vi "18_TimeTaggerNetwork_server.vi"(8 "error in (no error)":errorcluster) -> (0 "error out":errorcluster)   [LabVIEW 2014]
uses:
  SwabianInstruments.TimeTagger
panel:
  out "log messages":string
  out "test signal":bool[](array[boolean])
  out "Counter measurement":i32[][](graph)
  in  "stop":bool
  # "Run the program to set up a server on default port 41101.\n\nThis VI will switch on and off the internal test-signal on channels 1-4\nin a cyclic pattern. \n\nYou can use the VI 18_TimeTaggerNetwork_client.vi to connect to this\nserver and to repeat the measurement on the client side."
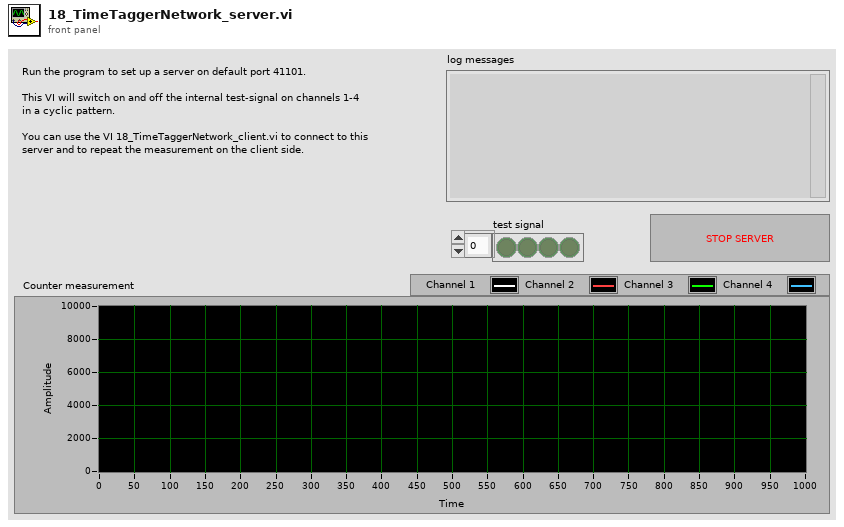
[diagram p1: front panel]
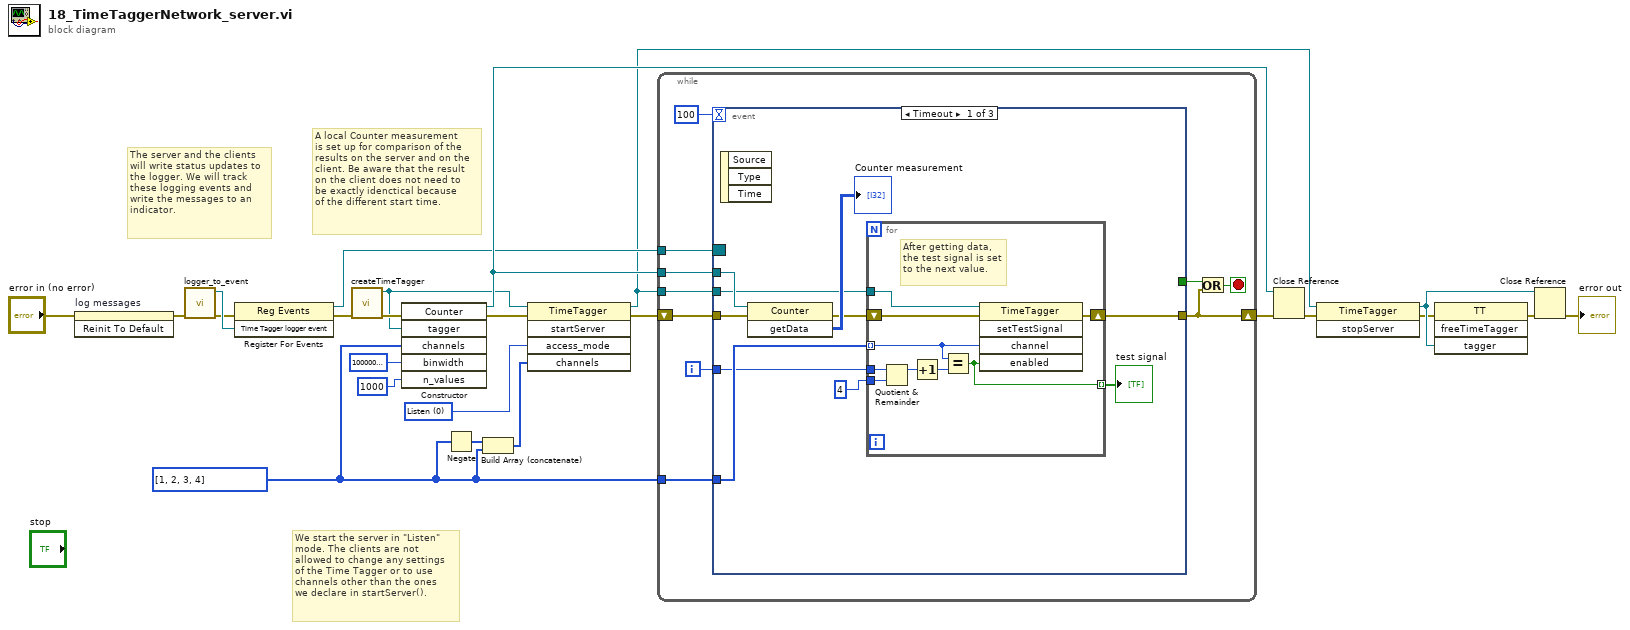
[diagram p0: block diagram]
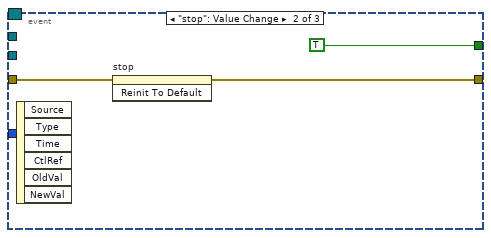
[diagram p2: hidden frame]
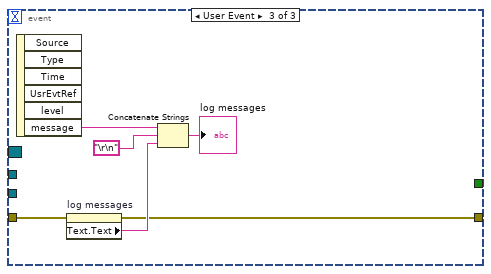
[diagram p3: hidden frame]
diagram:
  w14 = 0 items=["Listen", "Synchronous", "Control", "SynchronousControl"] ("access")
  w2 = i32[] [1, 2, 3, 4] ("channel")
  # "A local Counter measurement\nis set up for comparison of the\nresults on the server and on the\nclient. Be aware that the result\non the client does not need to\nbe exactly idenctical because\nof the different start time."
  # "The server and the clients\nwill write status updates to\nthe logger. We will track\nthese logging events and\nwrite the messages to an\nindicator."
  # "We start the server in \"Listen\"\nmode. The clients are not\nallowed to change any settings\nof the Time Tagger or to use\nchannels other than the ones\nwe declare in startServer()."
  n1 = invoke on="log messages" class="Str" method="Reinit To Default"(error in="error in (no error)") -> (error out=w6:errorcluster)  [unwired: 2 in, 2 out]
  n2 = call "logger_to_event.vi"("error in (no error)"=w6) -> ("error out"=w11:errorcluster, "Time Tagger logger event"=w13:refnum<user-event>)  [unwired: 9 in]
  n3 = register-events(error in=w11, w13) -> (reference out=w9:refnum<event-registration>, error out=w10:errorcluster)  [unwired: 1 in]
  n4 = call "createTimeTagger.vi"("error in (no error)"=w10) -> ("error out"=w16:errorcluster, "TimeTagger ref out"=w15:refnum<k24>)  [unwired: 9 in]
  n5 = constructor class="Counter"(error in=w16, "tagger"=w15, "channels"=w2, "binwidth"=i64 10000000000, "n_values"=1000) -> (reference out=w19:refnum<k24>, error out=w22:errorcluster)  [unwired: 2 in, 5 out]
  n6 = Negate(x=w2) -> (-x=w24:i32[])
  n7 = Build Array (concatenate)(w24, w2) -> (w23:i32[])
  n8 = invoke class="TimeTagger" method="startServer"(reference=w15, error in=w22, "access_mode"=w14, "channels"=w23) -> (reference out=w1:refnum<k24>, error out=w12:errorcluster)  [unwired: 1 in, 3 out]
  n9 = while {
    shift-right: [w28] -> w21
    shift-left: w12 -> [w34]
    tunnel: w19 -> [w33]
    tunnel: w9 -> [w27]
    tunnel: w2 -> [w26]
    tunnel: w1 -> [w25]
    i -> [w30]
    stop <- w29 stop-if-true
    n10 = event shown="[0] Timeout" {
      selector: w27 -> [_ _ _]
      dyn-events: _ -> [_ _ _]
      timeout: 100 -> [_ _ _]
      tunnel: w34 -> [w43 w56 w62]
      tunnel: [w40 w55 w57] -> w28
      tunnel: w33 -> [w44 _ _]
      tunnel: [_ TRUE _] -> w31
      tunnel: w30 -> [w37 _ _]
      tunnel: w26 -> [w39 _ _]
      tunnel: w25 -> [w38 _ _]
      event Timeout {
        n11 = event-data() -> ()  [unwired: 1 in, 3 out]
        n12 = invoke class="Counter" method="getData"(reference=w44, error in=w43) -> (error out=w41:errorcluster, "getData"=→"Counter measurement":i32[][])  [unwired: 1 in, 1 out]
        n13 = for {
          tunnel: w39 -> [w48] mode=indexing
          shift-right: [w52] -> w40
          shift-left: w41 -> [w53]
          tunnel: w38 -> [w51]
          tunnel: w37 -> [w50]
          tunnel: 4 ("y") -> [w49]
          tunnel: [w46] -> w35 mode=indexing
          # "After getting data,\nthe test signal is set\nto the next value."
          n14 = Quotient & Remainder(x=w50, y=w49) -> (x-y*floor(x/y)=w45:i32)  [unwired: 1 out]
          n15 = Increment(x=w45) -> (x+1=w47:i32)
          n16 = Equal?(x=w48, y=w47) -> (x = y?=w46:bool)
          n17 = invoke class="TimeTagger" method="setTestSignal"(reference=w51, error in=w53, "channel"=w48, "enabled"=w46) -> (error out=w52:errorcluster)  [unwired: 1 in, 4 out]
        }
        "test signal" <- w35
      }
      event "stop": Value Change {
        n18 = event-data() -> ()  [unwired: 1 in, 6 out]
        n19 = invoke on="stop" class="Bool" method="Reinit To Default"(error in=w56) -> (error out=w55:errorcluster)  [unwired: 2 in, 2 out]
      }
      event User Event {
        n20 = event-data() -> ("message"=w59:string)  [unwired: 1 in, 5 out]
        n21 = property on="log messages" class="Str"(error in=w62) -> (error out=w57:errorcluster, "Text.Text"=w61:string)  [unwired: 1 in, 1 out]
        n22 = Concatenate Strings(w59, "\r\n", w61) -> (→"log messages":string)
      }
    }
    n23 = Or(x=w31, y=w28) -> (x .or. y?=w29:bool)
  }
  n24 = Close Reference(reference=w19, error in (no error)=w21) -> (error out=w20:errorcluster)
  n25 = invoke class="TimeTagger" method="stopServer"(reference=w1, error in=w20) -> (reference out=w5:refnum<k24>, error out=w4:errorcluster)  [unwired: 1 in, 1 out]
  n26 = invoke class="TT" method="freeTimeTagger"(error in=w4, "tagger"=w5) -> (error out=w3:errorcluster)  [unwired: 2 in, 3 out]
  n27 = Close Reference(reference=w5, error in (no error)=w3) -> (error out=→"error out":errorcluster)
